vi "SwerveKinematics_ToTwst2d4.vi"(7 "in SWERVE_DRIVE_KINEMATICS":T4 {"SavedModuleStates"."Angle"."SIN" format="%13.4f"; "SavedModuleStates"."Angle"."COS" format="%13.4f"; "SavedModuleStates"."Angle"."VALUE" format="%13.4f"; "PrevCoR"."Y" format="%14.3f"; "PrevCoR"."X" format="%14.3f"; "Modules"."Y" format="%14.3f"; "Modules"."X" format="%14.3f"}, 8 "Wheel Delta 3":T1={"Distance"=0.0, "Angle"={"VALUE"=0.0, "COS"=1.0, "SIN"=0.0}} {"Angle"."SIN" format="%13.4f"; "Angle"."COS" format="%13.4f"; "Angle"."VALUE" format="%13.4f"}, 9 "Wheel Delta 2":T1={"Distance"=0.0, "Angle"={"VALUE"=0.0, "COS"=1.0, "SIN"=0.0}} {"Angle"."SIN" format="%13.4f"; "Angle"."COS" format="%13.4f"; "Angle"."VALUE" format="%13.4f"}, 10 "Wheel Delta 1":T1={"Distance"=0.0, "Angle"={"VALUE"=0.0, "COS"=1.0, "SIN"=0.0}} {"Angle"."SIN" format="%13.4f"; "Angle"."COS" format="%13.4f"; "Angle"."VALUE" format="%13.4f"}, 11 "Wheel Delta 0":T1={"Distance"=0.0, "Angle"={"VALUE"=0.0, "COS"=1.0, "SIN"=0.0}} {"Angle"."SIN" format="%13.4f"; "Angle"."COS" format="%13.4f"; "Angle"."VALUE" format="%13.4f"}) -> (1 "Error":bool, 3 "Twist2d":T3)   [LabVIEW 2019, in "Trajectory_Library.lvlib"]
doc: "Performs forward kinematics to return the resulting chassis state from the given module states. This method is often used for odometry -- determining the robot's position on the field using data from the real-world speed and angle of each module on the robot.\n\nParameters: \n - in Swerve Drive Kinematics - Swerve drive kinematics data structure\n - wheelDelta 0 - The latest change in position of the modules (as a SwerveModulePosition type) as measured from respective encoders and gyros. The order of the swerve module states should be same as passed into the constructor of this class.\n - wheelDelta 1 - Another wheel position \n - wheelDelta 2 - Another wheel position\n - wheelDelta 3 - Another wheel position\n\nReturns:\n - The resulting twist2d."
uses:
  Trajectory_Library.lvlib
  TypeDef/SWERVE_DRIVE_KINEMATICS.ctl
  <vilib>/Analysis/Matrix/Datatypes/RealMatrix.ctl
  TypeDef/TRANSLATION2D.ctl
  TypeDef/SWERVE_DRIVE_MODULE_STATE.ctl
  TypeDef/ROTATION2D.ctl
  TypeDef/TWIST2D.ctl
  TypeDef/SWERVE_DRIVE_MODULE_POSITION.ctl
  <vilib>/Analysis/Matrix/NI_Matrix.lvlib
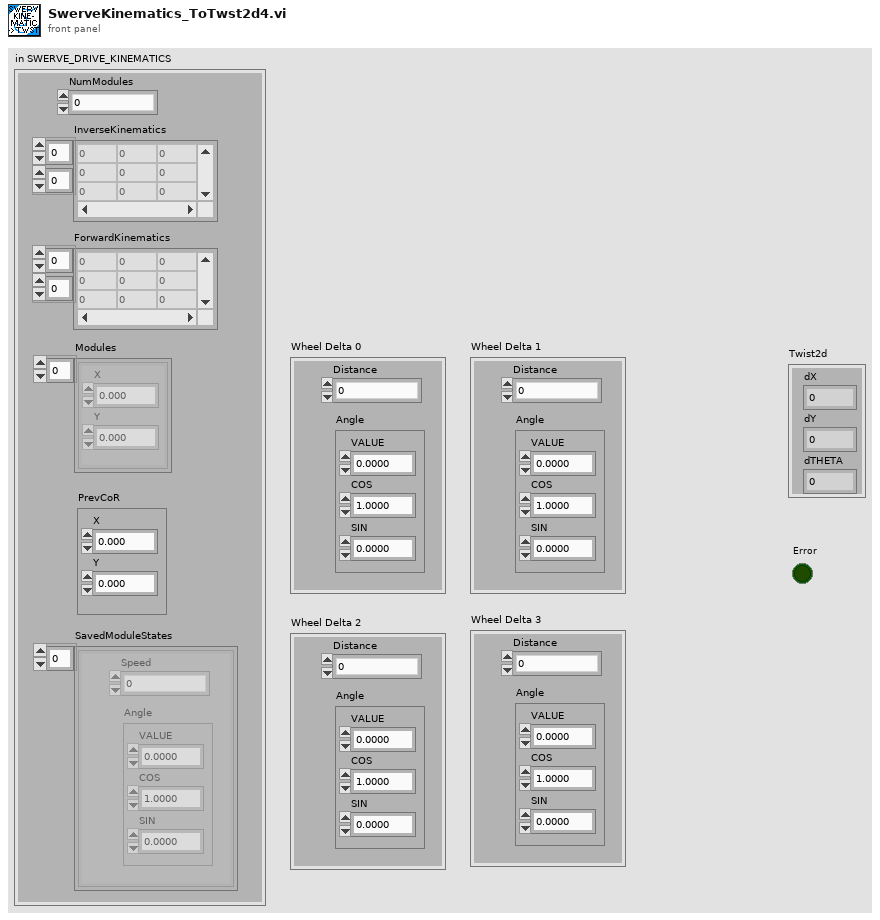
[diagram p1: front panel]
types:
  T1 = typedef "Trajectory_Library.lvlib/SWERVE_DRIVE_MODULE_POSITION.ctl" = cluster{"Distance":dbl, "Angle":T2}
  T2 = typedef "Trajectory_Library.lvlib/ROTATION2D.ctl" = cluster{"VALUE":dbl, "COS":dbl, "SIN":dbl}
  T3 = typedef "Trajectory_Library.lvlib/TWIST2D.ctl" = cluster{"dX":dbl, "dY":dbl, "dTHETA":dbl}
  T4 = typedef "Trajectory_Library.lvlib/SWERVE_DRIVE_KINEMATICS.ctl" = cluster{"NumModules":i32, "InverseKinematics":T5, "ForwardKinematics":T5, "Modules":T6[], "PrevCoR":T6, "SavedModuleStates":T7[]}
  T5 = typedef "NI_Matrix.lvlib/RealMatrix.ctl" = dbl[][]
  T6 = typedef "Trajectory_Library.lvlib/TRANSLATION2D.ctl" = cluster{"X":dbl, "Y":dbl}
  T7 = typedef "Trajectory_Library.lvlib/SWERVE_DRIVE_MODULE_STATE.ctl" = cluster{"Speed":dbl, "Angle":T2}
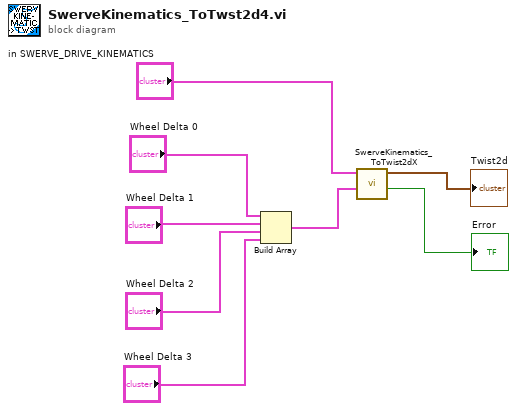
[diagram p0: block diagram]
diagram:
  n1 = Build Array("Wheel Delta 0", "Wheel Delta 1", "Wheel Delta 2", "Wheel Delta 3") -> (w3:T1[])
  n2 = call "SwerveKinematics_ToTwist2dX.vi"("WheelDeltas"=w3, "in SWERVE_DRIVE_KINEMATICS"="in SWERVE_DRIVE_KINEMATICS") -> ("Error"=→"Error":bool, "Twist2d"=→"Twist2d":T3)  [unwired: 8 in]
